vi "Database.GetTimeOfLatestParamChange.vi"(11 "TS":cluster{"TS":T1, "TP":T2[], "TV":T3[]}[](array[cluster]) {"TP"."value" format="%#.3f"; "TV"."minimum" format="%#.3f"; "TV"."maximum" format="%#.3f"}) -> (0 "Maxs":string[](array[string]), 1 "Mins":string[](array[string]), 2 "Params":string[](array[string]), 3 "Max":timestamp, 4 "VariantFileValues":cluster{string[], string[], string[]})   [LabVIEW 2016]
uses:
  ProdaNG/Controls/ProdaNG.TestStep.ctl
  ProdaNG/Controls/ProdaNG.TestStepParam.ctl
  ProdaNG/Controls/ProdaNG.TestValue.ctl
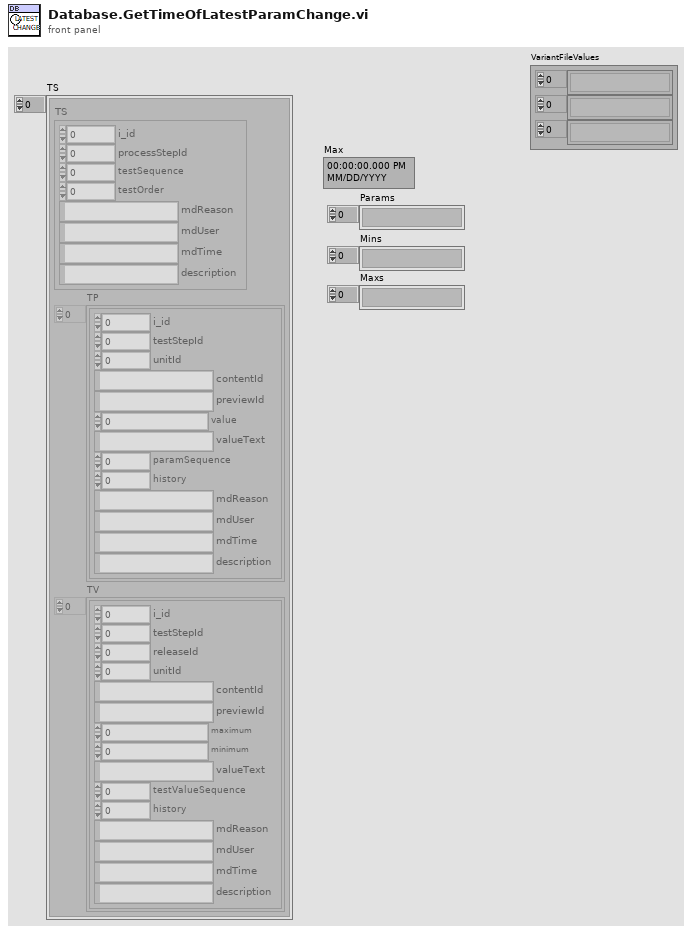
[diagram p1: front panel]
types:
  T1 = typedef "ProdaNG.TestStep.ctl" = cluster{"i_id":i32, "processStepId":i32, "testSequence":i32, "testOrder":i32, "mdReason":string, "mdUser":string, "mdTime":string, "description":string}
  T2 = typedef "ProdaNG.TestStepParam.ctl" = cluster{"i_id":i32, "testStepId":i32, "unitId":i32, "contentId":string, "previewId":string, "value":dbl, "valueText":string, "paramSequence":i32, "history":i32, "mdReason":string, "mdUser":string, "mdTime":string, "description":string}
  T3 = typedef "ProdaNG.TestValue.ctl" = cluster{"i_id":i32, "testStepId":i32, "releaseId":i32, "unitId":i32, "contentId":string, "previewId":string, "maximum":dbl, "minimum":dbl, "valueText":string, "testValueSequence":i32, "history":i32, "mdReason":string, "mdUser":string, "mdTime":string, "description":string}
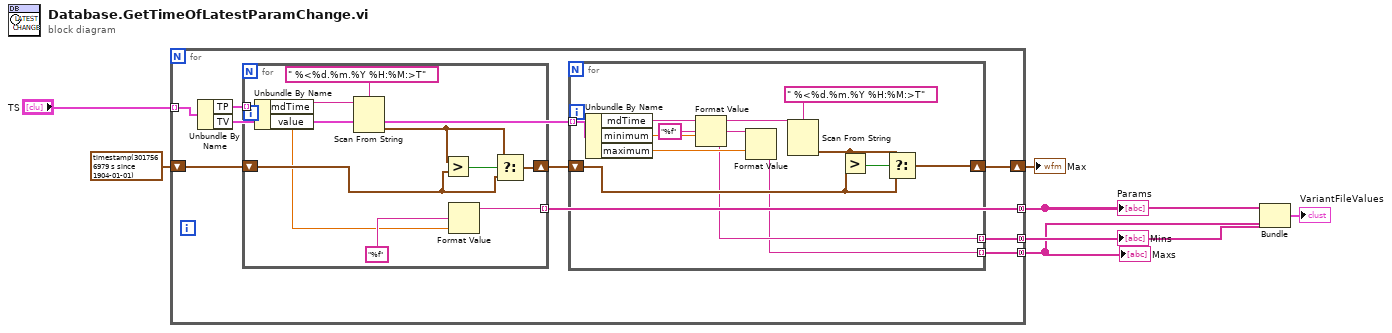
[diagram p0: block diagram]
diagram:
  n1 = for {
    tunnel: "TS" -> [w16] mode=indexing
    shift-right: [w11] -> w7
    shift-left: timestamp(3017566979 s since 1904-01-01) ("Max") -> [w14]
    tunnel: [w10] -> w4 mode=concatenating
    tunnel: [w9] -> w3 mode=concatenating
    tunnel: [w8] -> w2 mode=concatenating
    n2 = Unbundle By Name(w16) -> ("TP"=w15:T2[], "TV"=w13:T3[])
    n3 = for {
      tunnel: w15 -> [w38] mode=indexing
      shift-right: [w33] -> w12
      shift-left: w14 -> [w32]
      tunnel: [w29] -> w10 mode=indexing
      n4 = Unbundle By Name(w38) -> ("mdTime"=w36:string, "value"=w30:dbl)
      n5 = Scan From String(format string=" %<%d.%m.%Y %H:%M:>T", input string=w36) -> (output 1=w34:timestamp)  [unwired: 3 in, 3 out]
      n6 = Greater?(x=w34, y=w32) -> (0:w35:bool)
      n7 = Format Value(format string="%f", value (0)=w30) -> (output string=w29:string)  [unwired: 1 in]
      n8 = Select(t=w34, s=w35, f=w32) -> (s? t:f=w33:timestamp)
    }
    n9 = for {
      tunnel: w13 -> [w28] mode=indexing
      shift-right: [w22] -> w11
      shift-left: w12 -> [w24]
      tunnel: [w18] -> w9 mode=indexing
      tunnel: [w17] -> w8 mode=indexing
      w19 = "%f" ("format string")
      n10 = Unbundle By Name(w28) -> ("mdTime"=w27:string, "minimum"=w21:dbl, "maximum"=w20:dbl)
      n11 = Format Value(format string=w19, value (0)=w21) -> (output string=w18:string)  [unwired: 1 in]
      n12 = Format Value(format string=w19, value (0)=w20) -> (output string=w17:string)  [unwired: 1 in]
      n13 = Scan From String(format string=" %<%d.%m.%Y %H:%M:>T", input string=w27) -> (output 1=w23:timestamp)  [unwired: 3 in, 3 out]
      n14 = Greater?(x=w23, y=w24) -> (0:w25:bool)
      n15 = Select(t=w23, s=w25, f=w24) -> (s? t:f=w22:timestamp)
    }
  }
  "Max" <- w7
  "Params" <- w4
  "Mins" <- w3
  "Maxs" <- w2
  n16 = Bundle(w4, w3, w2) -> (→"VariantFileValues":cluster{string[], string[], string[]})  [unwired: 1 in]
